vi "Launch Preparation.vi"(8 "error in (no error)":errorcluster, 11 "AMS Gas in":refnum<class "AMS Gas.lvclass">) -> (0 "error out":errorcluster, 3 "AMS Gas out":refnum<class "AMS Gas.lvclass">)   [LabVIEW 2015, in "AMS UI.lvlib" / "AMS Gas.lvclass"]
uses:
  AMS Gas.lvclass
  <vilib>/ActorFramework/Actor/Actor.lvclass
  Preparation/Preparation.lvclass
  AMS Gas.lvclass/AMS Gas.ctl
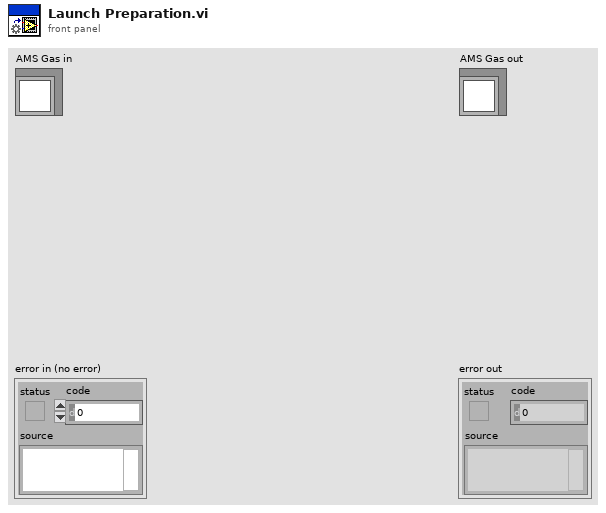
[diagram p1: front panel]
types:
  T1 = typedef "FP Control Refs Cluster.ctl" = cluster{"Liquid N Valve References":T2, "Main Line Valve Refs":T3, "Transfer Line Container":refnum<vi>, "Storage Containers":refnum<vi>[], "Sample Refs":T4, "Syringe Ctrl Refs ":T5, "Baratrons Chart":refnum<vi>, "Capillary Container":refnum<vi>, "Preparation Container":refnum<vi>, "Monkey Mode":refnum<vi>}
  T2 = typedef "Liquid N Valve Ref Cluster.ctl" = cluster{"Cold Bath H2O HV 100":refnum<vi>, "Cold Bath Cleaning HV 101":refnum<vi>, "Cold Bath Storage 1 HV 102":refnum<vi>, "Cold Bath Storage 2 HV 103":refnum<vi>, "Cold Bath Storage 3 HV 104":refnum<vi>, "Cold Bath Storage 4 HV 105":refnum<vi>, "Cold Bath Syringe HV 106":refnum<vi>, "Liquid N Master Valve HV 107":refnum<vi>}
  T3 = typedef "Main Line Valve Ref Cluster.ctl" = cluster{"Turbo Valve DV313":refnum<vi>, "Prep Line Valve 0 DV300":refnum<vi>, "Storage Valves":refnum<vi>[]}
  T4 = typedef "Sample Valve Refs.ctl" = cluster{"Valves":cluster{"Sample 5 DV318":refnum<vi>, "Sample 4 DV317":refnum<vi>, "Sample 3 DV316":refnum<vi>, "Sample 2 DV315":refnum<vi>, "Sample 1 DV314":refnum<vi>}, "Lines":cluster{"Sample 1":refnum<vi>, "Sample 2":refnum<vi>, "Sample 3":refnum<vi>, "Sample 4":refnum<vi>, "Sample 5":refnum<vi>}}
  T5 = typedef "Syringe Ctrl Refs.ctl" = cluster{"Syringe Home":refnum<vi>, "Syringe Freeze":refnum<vi>, "Syringe TC":refnum<vi>, "Syringe Container":refnum<vi>}
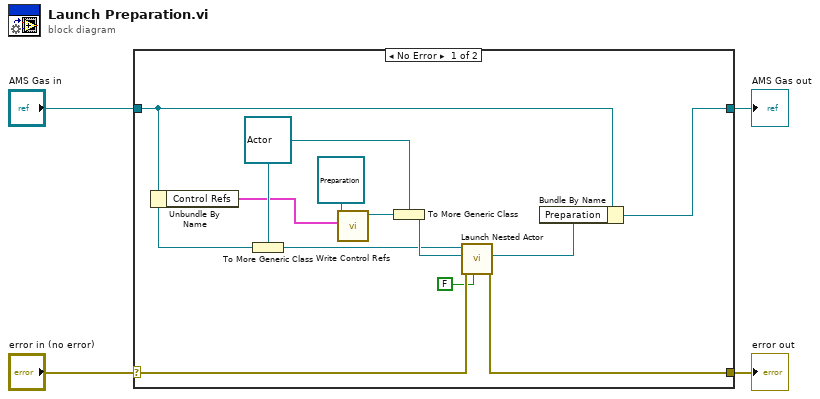
[diagram p0: block diagram]
diagram:
  n1 = case shown="No Error" "error in (no error)" {
    selector: "error in (no error)" -> [w14 w18]
    tunnel: [w13 w18] -> w3
    tunnel: "AMS Gas in" -> [w11 w17]
    tunnel: [w8 w17] -> w1
    frame No Error {
      w10 = refnum<class "Actor.lvclass"> refnum ("Actor")
      n2 = Unbundle By Name(w11) -> ("Control Refs"=w9:T1)
      n3 = To More Generic Class(target class=w10, reference=w11) -> (generic class reference=w6:refnum<class "Actor.lvclass">)
      n4 = call-dynamic "Write Control Refs.vi"("Control Refs"=w9, "AMS Gas Actor in"=refnum<class "Preparation.lvclass"> refnum ("Preparation.lvclass")) -> ("AMS Gas Actor out"=w16:refnum<class "Preparation.lvclass">)  [unwired: 9 in]
      n5 = To More Generic Class(target class=w10, reference=w16) -> (generic class reference=w7:refnum<class "Actor.lvclass">)
      n6 = call <vilib>:"Launch Nested Actor.vi"("Open Actor Core front panel? (F)"=FALSE, "error in (no error)"=w14, "Nested Actor"=w7, "Caller Actor in"=w6) -> ("error out"=w13:errorcluster, "Nested Actor's Enqueuer"=w15:refnum<class "Message Enqueuer.lvclass">)  [unwired: 5 in, 1 out]
      n7 = Bundle By Name(cluster=w11, "Preparation"=w15) -> (w8:refnum<class "AMS Gas.lvclass">)
    }
    frame Error {
    }
  }
  "error out" <- w3
  "AMS Gas out" <- w1
